vi "Find and Compile.vi"(8 "error in (no error)":errorcluster, 11 "Project Path":path) -> (0 "error out":errorcluster)   [LabVIEW 2015, in "HTML Help File Tools.lvlib"]
uses:
  HTML Help File Tools.lvlib
  Log FGV Operation Modes.ctl
  Error Location.ctl
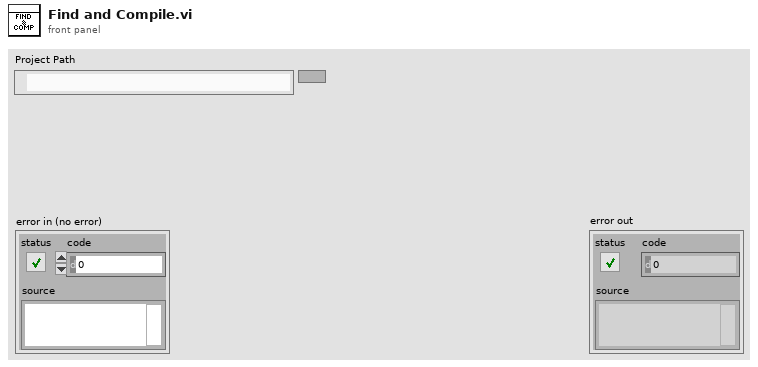
[diagram p1: front panel]
types:
  T1 = typedef "HTML Help File Tools.lvlib/Log FGV Operation Modes.ctl" = enum16{"Close", "Write", "Open File"}
  T2 = typedef "HTML Help File Tools.lvlib/Error Location.ctl" = enum16{"Delete tmp", "Compile HHP", "Find Install", "Create tmp", "Create HHP", "Find Help"}
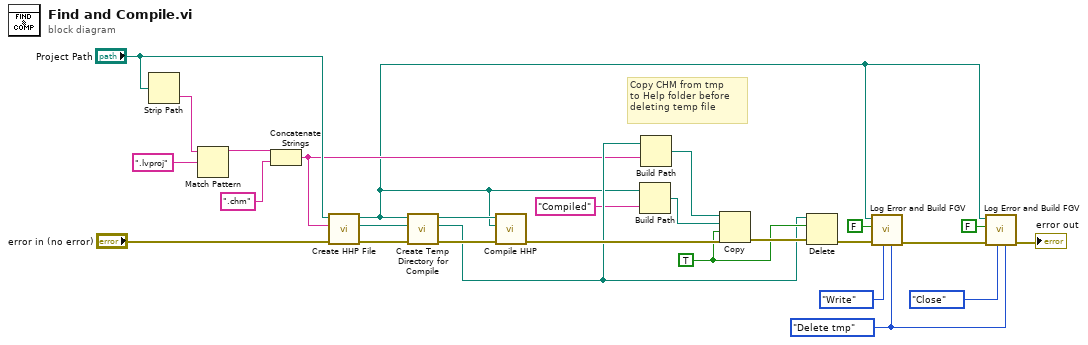
[diagram p0: block diagram]
diagram:
  w2 = Error_Location."Delete tmp" ("Error Location")
  w15 = TRUE ("entire hierarchy (F)")
  # "Copy CHM from tmp \nto Help folder before \ndeleting temp file"
  n1 = Strip Path(path="Project Path") -> (name=w24:string)  [unwired: 1 out]
  n2 = Match Pattern(string=w24, regular expression=".lvproj") -> (before substring=w25:string)  [unwired: 1 in, 3 out]
  n3 = Concatenate Strings(w25, ".chm" ("regular expression")) -> (w12:string)
  n4 = call "Create HHP File.vi"("error in (no error)"="error in (no error)", "Name of Compiled File"=w12, "Project Path"="Project Path") -> ("error out"=w21:errorcluster, ".hhp file path"=w19:path, "Help Documentation Path"=w1:path)  [unwired: 6 in]
  n5 = call "Create Temp Directory for Compile.vi"("error in (no error)"=w21, ".hhp file path"=w19, "Help Path"=w1) -> ("error out"=w20:errorcluster, "temp directory"=w14:path, "temp .hhp path"=w18:path)  [unwired: 6 in]
  n6 = call "Compile HHP.vi"("error in (no error)"=w20, "Help Path"=w1, "temp .hhp path"=w18) -> ("error out"=w17:errorcluster)  [unwired: 6 in, 2 out]
  n7 = Build Path(base path=w1, name or relative path="Compiled") -> (appended path=w10:path)
  n8 = Build Path(base path=w14, name or relative path=w12) -> (appended path=w13:path)
  n9 = Copy(8:w17, 9:w15, 10:w10, 11:w13) -> (0:w16:errorcluster)  [unwired: 1 in, 2 out]
  n10 = Delete(path (use dialog)=w14, entire hierarchy (F)=w15, error in=w16) -> (error out=w9:errorcluster)  [unwired: 2 in, 2 out]
  n11 = call "Log Error and Build FGV.vi"("Error Location"=w2, "Operation Mode"=Log_FGV_Operation_Modes."Write", "error in"=w9, "Log Build Output?"=FALSE, "Help Documentation Path"=w1) -> ("error out"=w6:errorcluster)  [unwired: 6 in]
  n12 = call "Log Error and Build FGV.vi"("Error Location"=w2, "Operation Mode"=Log_FGV_Operation_Modes."Close", "error in"=w6, "Log Build Output?"=FALSE, "Help Documentation Path"=w1) -> ("error out"=→"error out":errorcluster)  [unwired: 6 in]
